vi "timer_test.vi"() -> ()   [LabVIEW 2020]
panel:
  in  "Boolean 2":bool
  in  "Boolean":bool
  out "Present (s)":dbl
  in  "stop":bool
  out "Elapsed Time (s)":dbl
  out "Elapsed Time Text":string
  out "Present Text":string
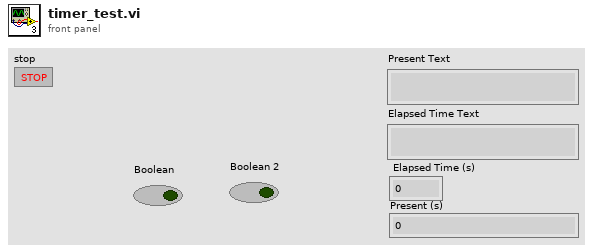
[diagram p1: front panel]
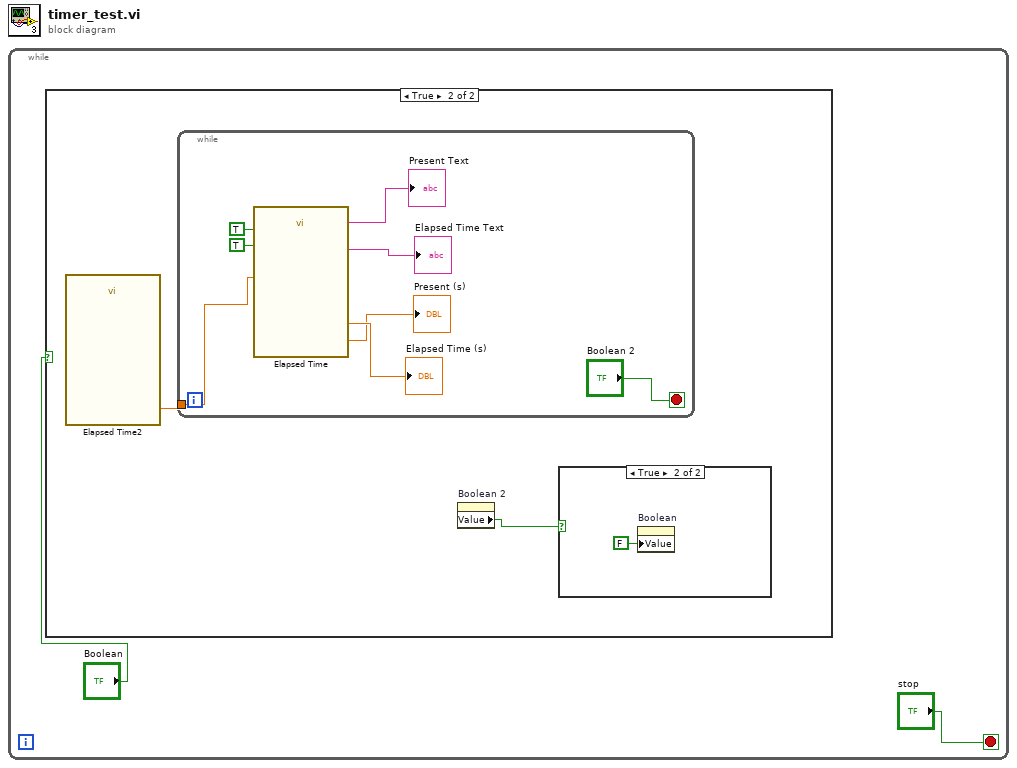
[diagram p0: block diagram]
diagram:
  n1 = while {
    stop <- "stop" stop-if-true
    n2 = case shown="True" "Boolean" {
      frame False {
      }
      frame True {
        n3 = call "Elapsed Time2"() -> ("Present (s)"=w3:dbl)  [unwired: 12 in, 7 out]
        n4 = while {
          tunnel: w3 -> [w6]
          stop <- "Boolean 2" stop-if-true
          n5 = call "Elapsed Time"("Reset"=TRUE, "Auto Reset"=TRUE, "Set Start Time (s)"=w6) -> ("Present (s)"=→"Present (s)":dbl, "Present Text"=→"Present Text":string, "Elapsed Time (s)"=→"Elapsed Time (s)":dbl, "Elapsed Time Text"=→"Elapsed Time Text":string)  [unwired: 9 in, 4 out]
        }
        n6 = property on="Boolean 2" class="Bool (strict)"() -> ("Value"=w4:bool)  [unwired: 2 in, 2 out]
        n7 = case shown="True" w4 {
          frame False {
          }
          frame True {
            n8 = property on="Boolean" class="Bool (strict)"("Value"=FALSE ("Boolean")) -> ()  [unwired: 2 in, 2 out]
          }
        }
      }
    }
  }
